vi "_Remote Program Oscil.vi"(1 "error in (no error)":errorcluster) -> (0 "error out":errorcluster)   [LabVIEW 2015]
uses:
  Type/_RT Command.ctl
  Configuration/_Global Configuration.vi
panel:
  out "Array":string[](array[string])
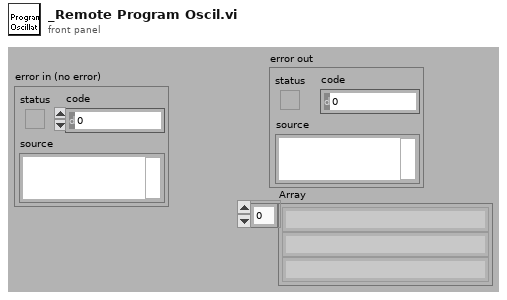
[diagram p1: front panel]
types:
  T1 = typedef "_RT Instrument 2.ctl" = cluster{"Table":T2[], "Instrument":string[]}
  T2 = typedef "_RT Configuration 2.ctl" = cluster{"Name":string, "Ch#":u8, "Min":dbl, "Max":dbl, "Def+":dbl, "Def-":dbl, "Offset":dbl, "Slope":dbl, "Type":u8, "Description":string, "SettleT":dbl}
  T3 = typedef "_RT Command.ctl" = enum16{"Start", "Stop", "Runtime Update", "Get Data", "Get Info", "Get Status", "Get Param", "Get Config", "Get Table", "Read ADC", "Set Oscillator", "Update Config", "Update Table", "Set All Pol", "Set Pol and DC", "Set Max Mass", "Toggle RP", "Toggle EL", "Set PIC", "Initialize Turbo", "Send Turbo Comm", "Close Turbo", "P1", "P2", "P3", "Send Serial", "Set LC Out", "Get LC In", "Read VAC", "Test Table", "Toggle Power", "Get Startup", "Set Startup", "Get ADC Table", "Set ADC Table", "Get Brief Status", "Get Detail Status", "Auxiliary Update", "Set CC Logics", "Set CC Input Logics", "Ignore Error"}
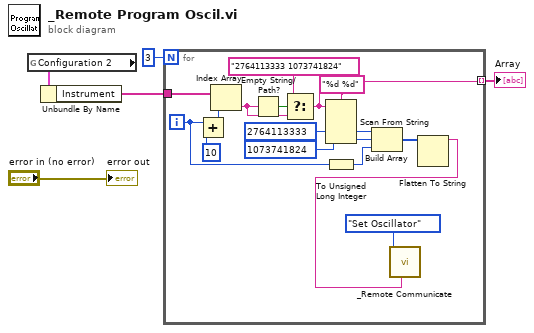
[diagram p0: block diagram]
diagram:
  n1 = global read "_Global Configuration.vi" "Configuration 2"() -> (w3:T1)
  n2 = Unbundle By Name(w3) -> ("Instrument"=w2:string[])
  n3 = for {
    N: 3 -> [_]
    tunnel: w2 -> [w22]
    tunnel: [w6] -> w1 mode=indexing
    i -> [w11]
    n4 = Add(x=w11, y=10) -> (x+y=w20:i32)
    n5 = Index Array(array=w22, index=w20) -> (element=w18:string)
    n6 = Empty String/Path?(string/path=w18) -> (empty?=w19:bool)
    n7 = Select(t="2764113333 1073741824", s=w19, f=w18) -> (s? t:f=w6:string)
    n8 = Scan From String(format string="%d %d", input string=w6, default 1=u32 2764113333 ("default value 1"), default 2=u32 1073741824 ("default value 1")) -> (output 1=w13:u32, output 2=w12:u32)  [unwired: 2 in, 3 out]
    n9 = To Unsigned Long Integer(number=w11) -> (unsigned 32bit integer=w10:u32)
    n10 = Build Array(w13, w12, w10) -> (w9:u32[])
    n11 = Flatten To String(anything=w9) -> (data string=w8:string)  [unwired: 1 in, 4 out]
    n12 = call "_Remote Communicate.vi"("String"=w8, "Command"=_RT_Command."Set Oscillator") -> ()  [unwired: 4 in, 4 out]
  }
  "Array" <- w1
  "error out" <- "error in (no error)"
